vi "Untitled 101.vi"() -> ()   [LabVIEW 2010]
uses:
  <vilib>/NXT/Block Support/NXT_InputPort.ctl
  <vilib>/NXT/Subs/MotorOutput.ctl
  <vilib>/NXT/Dual Mode Library/Motors/MotorOn.vi
  <vilib>/NXT/Dual Mode Library/Sensors/Sonar_cm.vi
  <vilib>/NXT/Dual Mode Library/Motors/MotorReverse.vi
panel:
  in  "Slide 2":dbl(slide) scale=0.0..60.0
  out "Slide":dbl(slide) scale=0.0..60.0
  in  "stop":bool
  in  "Output Port (All Ports)":T1=3 items=["Port A", "Port B", "Port C", "All Ports"]
  in  "Power (75)":i32=75
  out "Distance (cm)":i16
  in  "Port (Port 4)":T2=3 items=["Port 1", "Port 2", "Port 3", "Port 4"]
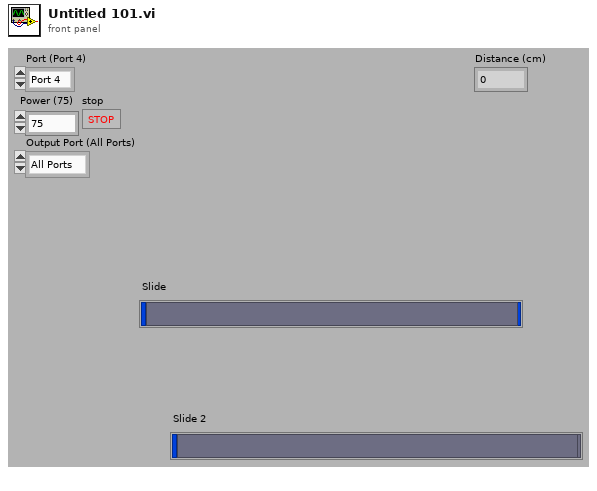
[diagram p1: front panel]
types:
  T1 = typedef "MotorOutput.ctl" = u8
  T2 = typedef "NXT_InputPort.ctl" = u8
  T3 = typedef "LVHSConnector.ctl" = cluster{"error":errorcluster, "address":string, "NXT #":i32, "Show Error":bool, "Connection":u16}
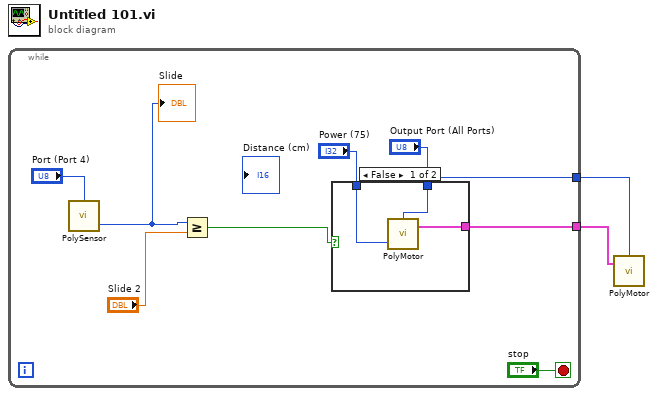
[diagram p0: block diagram]
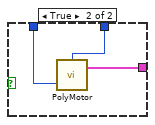
[diagram p2: hidden frame]
diagram:
  n1 = while {
    tunnel: ["Output Port (All Ports)"] -> w2
    tunnel: [w3] -> w1
    stop <- "stop" stop-if-true
    n2 = call-poly <vilib>:"PolySensor.vi"("Port (Port 4)"="Port (Port 4)") -> ("Distance (cm)"=w5:i16)  [unwired: 2 in, 1 out]
    "Slide" <- w5
    n3 = Greater Or Equal?(x=w5, y="Slide 2") -> (x >= y?=w9:bool)
    n4 = case shown="False" w9 {
      tunnel: "Power (75)" -> [w12 w15]
      tunnel: "Output Port (All Ports)" -> [w13 w16]
      tunnel: [w11 w14] -> w3
      frame False {
        n5 = call-poly <vilib>:"PolyMotor.vi"("Power (75)"=w12, "Output Port (All Ports)"=w13) -> ("NXT"=w11:T3)  [unwired: 2 in]
      }
      frame True {
        n6 = call-poly <vilib>:"PolyMotor.vi"("Power (75)"=w15, "Output Port (All Ports)"=w16) -> ("NXT"=w14:T3)  [unwired: 2 in]
      }
    }
  }
  n7 = call-poly <vilib>:"PolyMotor.vi"("NXT"=w1, "Output Port (All Ports)"=w2) -> ()  [unwired: 2 in, 1 out]
